vi "Next Step.vi"(8 "error in (no error)":errorcluster, 11 "Translation Stage in":refnum<class "Translation Stage.lvclass">) -> (0 "error out":errorcluster, 1 "Current Step":u32, 2 "Current Position":dbl, 3 "Translation Stage out":refnum<class "Translation Stage.lvclass">)   [LabVIEW 2009, in "Translation Stage.lvclass"]
uses:
  Translation Stage.lvclass
  Scanner/Scanner.lvclass
  Global/GPIB Numbers.vi
  Translation Stage.lvclass/Translation Stage.ctl
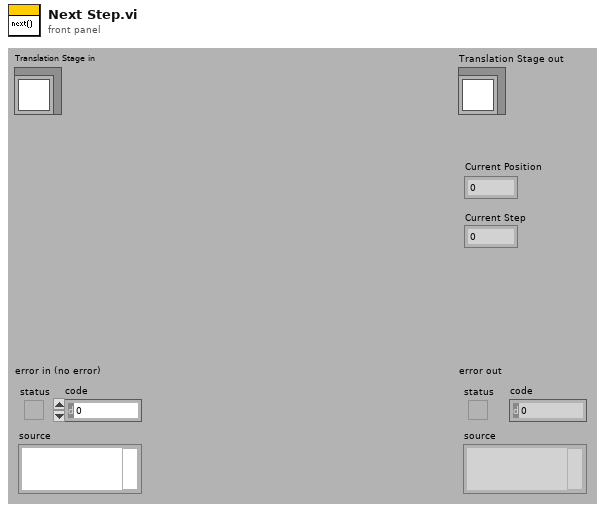
[diagram p1: front panel]
types:
  T1 = typedef "GPIB Type Def.ctl" = cluster{"Name":string, "bus":dbl, "GPIB":dbl, "GPIB as string":string, "byte":i32, "VISA Resource Name":refnum<visa-resource-name>}
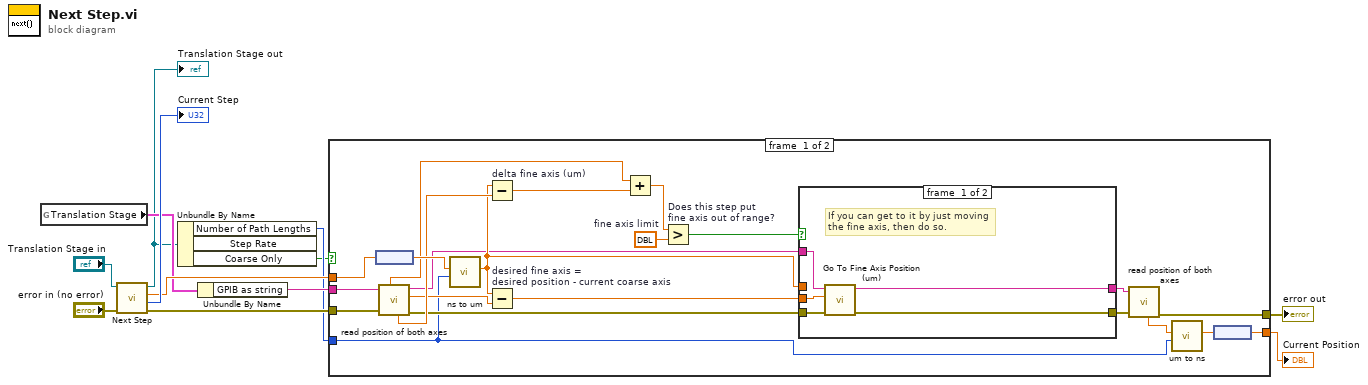
[diagram p0: block diagram]
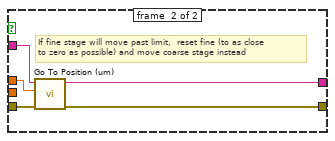
[diagram p2: hidden frame]
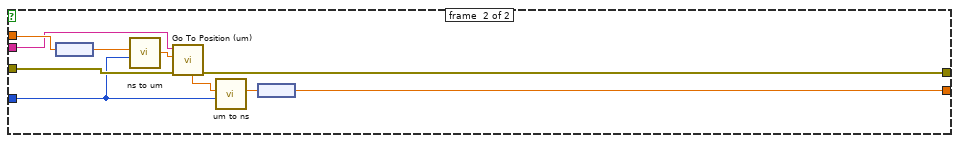
[diagram p3: hidden frame]
diagram:
  n1 = global read "GPIB Numbers.vi" "Translation Stage"() -> (w5:T1)
  n2 = call-parent "Next Step.vi"("error in (no error)"="error in (no error)", "Scanner in"="Translation Stage in") -> ("error out"=w8:errorcluster, "Current Step"=→"Current Step":u32, "Current Position"=w9:dbl, "Scanner out"=w3:refnum<class "Translation Stage.lvclass">)  [unwired: 6 out]
  "Translation Stage out" <- w3
  n3 = Unbundle By Name(w3) -> ("Number of Path Lengths"=w2:i32, "Coarse Only"=w1:bool)  [unwired: 1 out]
  n4 = Unbundle By Name(w5) -> ("GPIB as string"=w4:string)
  n5 = case shown="True" w1 {
    tunnel: w9 -> [w33 w54]
    tunnel: w8 -> [w32 w50]
    tunnel: [w26 w45] -> w7
    tunnel: [w22 w46] -> w6
    tunnel: w2 -> [w13 w48]
    tunnel: w4 -> [w17 w51]
    frame #0 {
      w29 = ext[unit] 0.045  # fine axis limit
      n6 = node(w33) -> (w34:dbl[unit])
      n7 = call "read position of both axes.vi"("GPIB # (in): def. 6"=w17, "error in (no error)"=w32) -> ("fine axis (um)"=w14:ext[unit], "GPIB # (out)"=w16:string, "coarse axis (um)"=w19:ext[unit], "combined position (um)"=w31:ext[unit], "error out"=w27:errorcluster)  [unwired: 4 out]
      n8 = call "ns to um.vi"("number of path lengths (default: 2)"=w13, "position (ns)"=w34) -> ("position (microns)"=w20:dbl[unit])  [unwired: 9 out]
      n9 = Subtract "delta fine axis (um)"(x=w20, y=w31) -> (x-y=w21:ext[unit])
      n10 = Subtract "desired fine axis = \ndesired position - current coarse axis"(x=w20, y=w19) -> (x-y=w18:ext[unit])
      n11 = Add(x=w14, y=w21) -> (x+y=w30:ext[unit])
      n12 = Greater? "Does this step put\nfine axis out of range?"(x=w30, y=w29) -> (0:w28:bool)
      n13 = case shown="True" w28 {
        tunnel: w20 -> [_ w44]
        tunnel: w27 -> [w38 w43]
        tunnel: [w37 w42] -> w25
        tunnel: w18 -> [w39 _]
        tunnel: w16 -> [w36 w41]
        tunnel: [w35 w40] -> w15
        frame #0 {
          # "If you can get to it by just moving \nthe fine axis, then do so."
          n14 = call "Go To Fine Axis Position (um).vi"("error in"=w38, "Fine Axis Position (um)"=w39, "GPIB # (in): def. 6"=w36) -> ("error out"=w37:errorcluster, "GPIB # (out)"=w35:string)  [unwired: 7 out]
        }
        frame #1 {
          # "If fine stage will move past limit,  reset fine (to as close \nto zero as possible) and move coarse stage instead"
          n15 = call "Go To Position (um).vi"("error in (no error)"=w43, "Position (um)"=w44, "GPIB # (in): def. 6"=w41) -> ("error out"=w42:errorcluster, "GPIB # (out)"=w40:string)  [unwired: 7 out]
        }
      }
      n16 = call "read position of both axes.vi"("GPIB # (in): def. 6"=w15, "error in (no error)"=w25) -> ("combined position (um)"=w24:ext[unit], "error out"=w26:errorcluster)  [unwired: 7 out]
      n17 = call "um to ns.vi"("# of path lengths (def.: 2)"=w13, "position (microns)"=w24) -> ("position (ns)"=w23:dbl[unit])  [unwired: 9 out]
      n18 = node(w23) -> (w22:dbl)
    }
    frame #1 {
      n19 = node(w54) -> (w53:dbl[unit])
      n20 = call "ns to um.vi"("number of path lengths (default: 2)"=w48, "position (ns)"=w53) -> ("position (microns)"=w52:dbl[unit])  [unwired: 9 out]
      n21 = call "Go To Position (um).vi"("error in (no error)"=w50, "Position (um)"=w52, "GPIB # (in): def. 6"=w51) -> ("error out"=w45:errorcluster, "combined position (um)"=w49:ext[unit])  [unwired: 7 out]
      n22 = call "um to ns.vi"("# of path lengths (def.: 2)"=w48, "position (microns)"=w49) -> ("position (ns)"=w47:dbl[unit])  [unwired: 9 out]
      n23 = node(w47) -> (w46:dbl)
    }
  }
  "error out" <- w7
  "Current Position" <- w6
